vi "Actor Core.vi"(8 "error in":errorcluster caption="错误输入", 11 "客户端代理者 in":refnum<class "客户端代理者.lvclass"> caption="操作者输入") -> (0 "error out":errorcluster caption="错误输出", 3 "Actor out":refnum<class "Actor.lvclass"> caption="操作者输出")   [LabVIEW 2015, in "客户端代理者.lvlib" / "客户端代理者.lvclass"]
doc: "(<B>文件名</B>: Actor Framework.lvlib:Actor.lvclass:Actor Core.vi)\n\n接收发送至操作者的消息，响应消息并处理可能导致操作者关闭的错误。\n\n子孙类重写该VI，使操作者完成特定的任务。使用调用父方法节点实现重写。"
uses:
  <vilib>/ActorFramework/Actor/Actor.lvclass
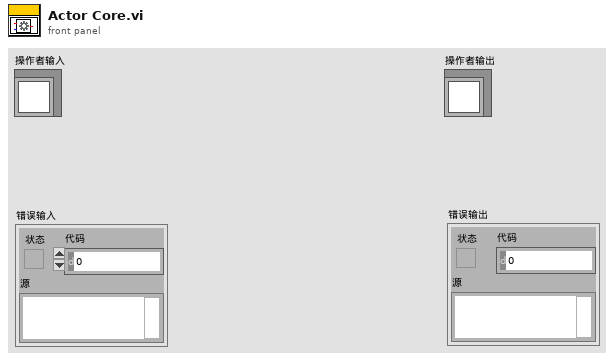
[diagram p1: front panel]
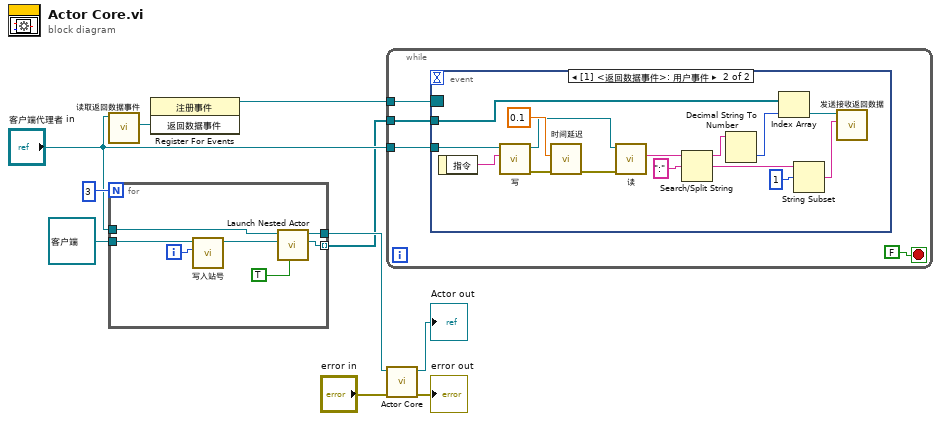
[diagram p0: block diagram]
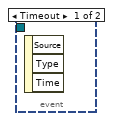
[diagram p2: hidden frame]
diagram:
  n1 = call-dynamic "读取返回数据事件.vi"("通讯输入"="客户端代理者 in") -> ("返回数据事件"=w7:refnum<user-event>)  [unwired: 8 in, 2 out]
  n2 = for {
    N: 3 -> [_]
    tunnel: refnum<class "客户端.lvclass"> refnum ("客户端操作者.lvlib:客户端.lvclass") -> [w17]
    tunnel: "客户端代理者 in" -> [w15]
    tunnel: [w12] -> w4
    tunnel: [w11] -> w1 mode=indexing
    i -> [w16]
    n3 = call-dynamic "写入站号.vi"("站号"=w16, "客户端输入"=w17) -> ("客户端输出"=w14:refnum<class "客户端.lvclass">)  [unwired: 8 in, 1 out]
    n4 = call <vilib>:"Launch Nested Actor.vi"("Open Actor Core front panel? (F)"=TRUE, "Nested Actor"=w14, "Caller Actor in"=w15) -> ("Nested Actor's Enqueuer"=w11:refnum<class "Message Enqueuer.lvclass">, "Caller Actor out"=w12:refnum<class "客户端代理者.lvclass">)  [unwired: 6 in, 1 out]
  }
  n5 = register-events(w7) -> (reference out=w6:refnum<event-registration>)  [unwired: 2 in, 1 out]
  n6 = while {
    tunnel: w6 -> [w20]
    tunnel: "客户端代理者 in" -> [w19]
    tunnel: w1 -> [w18]
    stop <- FALSE stop-if-true
    n7 = event shown="[1] <返回数据事件>: 用户事件" {
      selector: w20 -> [_ _]
      dyn-events: _ -> [_ _]
      timeout: _ -> [_ _]
      tunnel: w19 -> [_ w31]
      tunnel: w18 -> [_ w27]
      event Timeout {
        n8 = event-data() -> ()  [unwired: 1 in, 3 out]
      }
      event User Event {
        n9 = event-data() -> ("指令"=w35:string)  [unwired: 1 in]
        n10 = call-dynamic "写.vi"("写入缓冲区"=w35, "通讯 输入"=w31) -> ("error out"=w34:errorcluster, "通讯 输出"=w32:refnum<class "客户端代理者.lvclass">)  [unwired: 8 in]
        n11 = call "时间延迟"("error in (no error)"=w34, "Delay Time (s)"=0.1) -> ("error out"=w33:errorcluster)  [unwired: 9 in]
        n12 = call-dynamic "读.vi"("error in (no error)"=w33, "通讯 输入"=w32) -> ("读取缓冲区"=w22:string)  [unwired: 7 in, 2 out]
        n13 = Search/Split String(string=w22, search string/char (-)=":") -> (substring before match=w29:string, match + rest of string=w25:string)  [unwired: 1 in, 1 out]
        n14 = Decimal String To Number(string=w29) -> (number=w28:i32)  [unwired: 2 in, 1 out]
        n15 = Index Array(array=w27, index=w28) -> (element=w26:refnum<class "Message Enqueuer.lvclass">)
        n16 = String Subset(string=w25, offset (0)=1 ("偏移量(0)")) -> (substring=w23:string)  [unwired: 1 in]
        n17 = call "发送接收返回数据.vi"("返回的数据"=w23, "Message Enqueuer"=w26) -> ()  [unwired: 8 in, 2 out]
      }
    }
  }
  n18 = call-parent "Actor Core.vi"("error in"="error in", "Actor in"=w4) -> ("error out"=→"error out":errorcluster, "Actor out"=→"Actor out":refnum<class "Actor.lvclass">)  [unwired: 8 in]
